vi "Read Keys.vi"(8 "error in (no error)":errorcluster, 11 "Section in":refnum<class "Section.lvclass">) -> (0 "error out":errorcluster, 2 "Keys":cluster{"Name":string, "Value":string}[](array[cluster]), 3 "Section out":refnum<class "Section.lvclass">)   [LabVIEW 2013, in "Configuration.lvlib" / "Section.lvclass"]
doc: "Thi VI returns an array of key/values pairs of section.\n\nPublic dynamic dispatch VI to be overwritten by derived classes."
uses:
  Section.lvclass
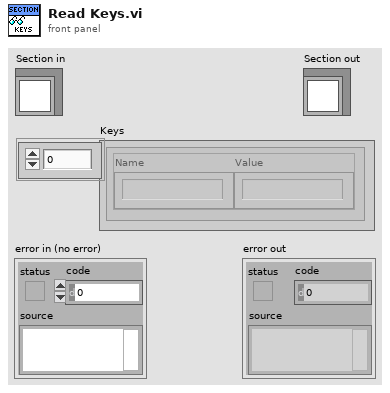
[diagram p1: front panel]
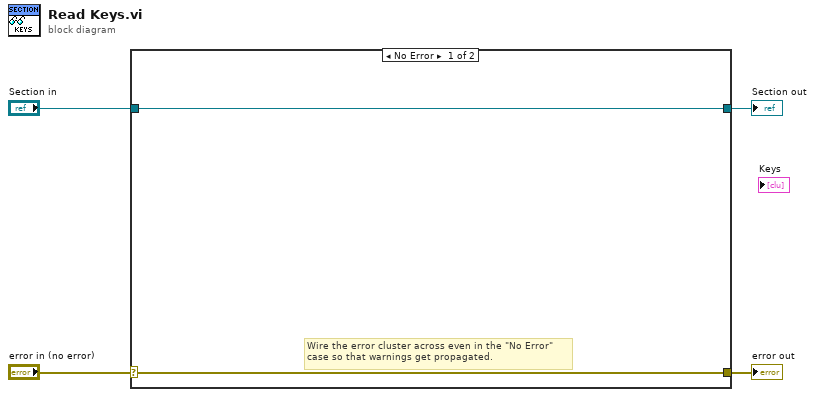
[diagram p0: block diagram]
diagram:
  n1 = case shown="No Error" "error in (no error)" {
    selector: "error in (no error)" -> [w5 w8]
    tunnel: [w5 w8] -> w3
    tunnel: [w6 w7] -> w1
    tunnel: "Section in" -> [w6 w7]
    frame No Error {
      # "Wire the error cluster across even in the \"No Error\"\ncase so that warnings get propagated."
    }
    frame Error {
    }
  }
  "error out" <- w3
  "Section out" <- w1
